vi "Cluster-Unbundle & Bundle.vi"() -> ()   [LabVIEW 2016]
panel:
  out "Cluster 2":T1
  out "Boolean":bool
  out "String":string
  out "Numeric":dbl
  in  "Cluster":T1
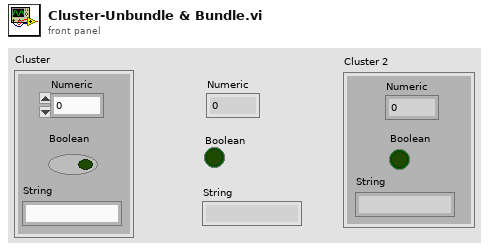
[diagram p1: front panel]
types:
  T1 = cluster{"Numeric":dbl, "Boolean":bool, "String":string}
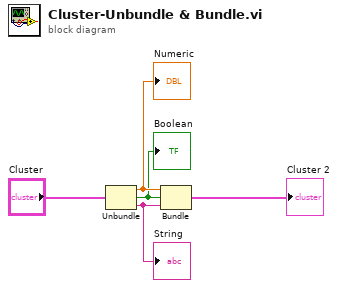
[diagram p0: block diagram]
diagram:
  n1 = Unbundle("Cluster") -> ("Numeric"=w3:dbl, "Boolean"=w2:bool, "String"=w1:string)
  "Numeric" <- w3
  "String" <- w1
  "Boolean" <- w2
  n2 = Bundle("Numeric"=w3, "Boolean"=w2, "String"=w1) -> (→"Cluster 2":T1)  [unwired: 1 in]
